vi "BAM Generation Create New TP Connection.vi"(5 "Data to Send":T1 {"Identifier" format="%08x"}, 11 "error in (no error)":errorcluster) -> (4 "Connection Cluster":T2 {"Packets"."Identifier" format="%08x"}, 6 "Connection Management Packet":T1 {"Identifier" format="%08x"}, 15 "error out":errorcluster)   [LabVIEW 2015, in "J1939 Addon Engine.lvlib"]
uses:
  J1939 Addon Engine.lvlib
  Types/BAM Generation Connection Cluster.ctl
  Shared/J1939 Utilities/Types/CAN Outgoing Message Cluster.ctl
  Shared/J1939 Utilities/SubVIs/TP.CM BAM.vi
  Shared/J1939 Utilities/SubVIs/TP.DT.vi
  Shared/J1939 Utilities/SubVIs/Convert CAN Arb ID to J1939 ID.vi
  Shared/J1939 Utilities/SubVIs/Convert J1939 ID to CAN Arb ID.vi
  Shared/J1939 Utilities/J1939 Utilities.lvlib
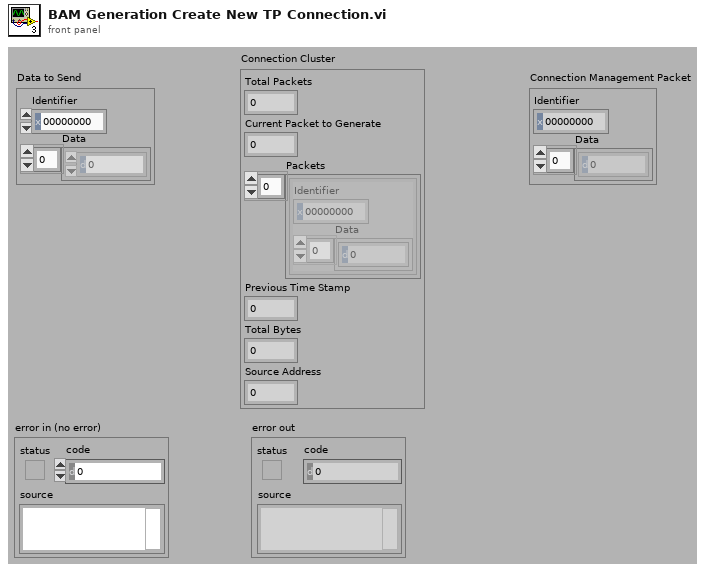
[diagram p1: front panel]
types:
  T1 = typedef "J1939 Addon Shared.lvlib/J1939 Utilities.lvlib/CAN Outgoing Message Cluster.ctl" = cluster{"Identifier":u32, "Data":u8[]}
  T2 = typedef "J1939 Addon Engine.lvlib/BAM Generation Connection Cluster.ctl" = cluster{"Total Packets":u8, "Current Packet to Generate":u8, "Packets":T1[], "Previous Time Stamp":u32, "Total Bytes":u16, "Source Address":u8}
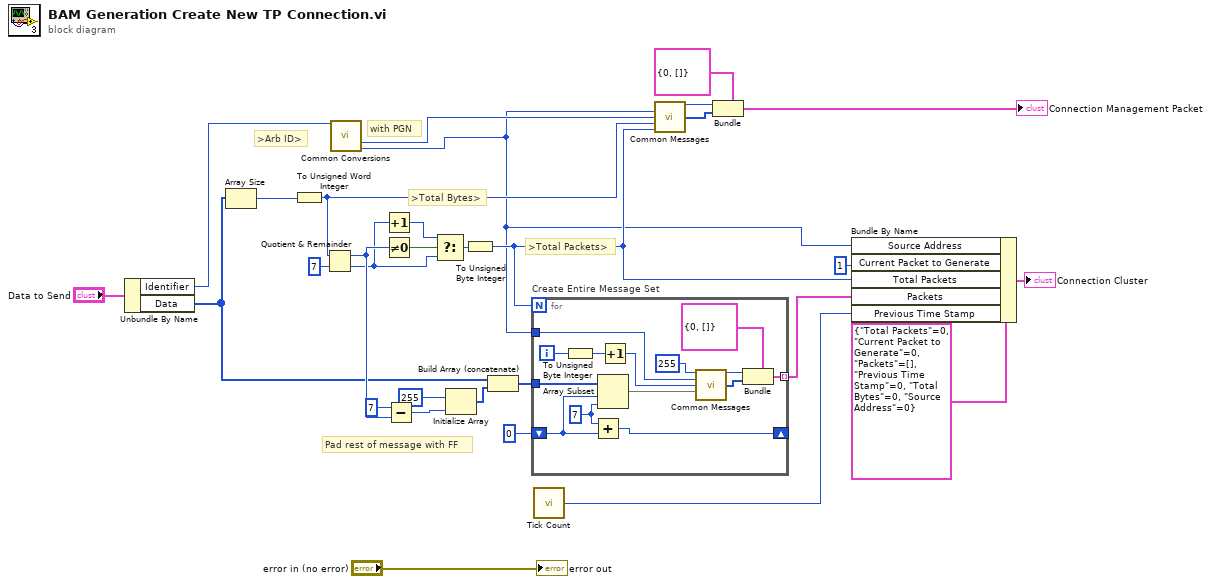
[diagram p0: block diagram]
diagram:
  # "Pad rest of message with FF"
  # ">Arb ID>"
  # "with PGN"
  # ">Total Packets>"
  # ">Total Bytes>"
  n1 = Unbundle By Name("Data to Send") -> ("Identifier"=w3:u32, "Data"=w5:u8[])
  n2 = Array Size(array=w5) -> (size(s)=w6:i32)
  n3 = To Unsigned Word Integer(number=w6) -> (unsigned 16bit integer=w12:u16)
  n4 = Quotient & Remainder(x=w12, y=u16 7) -> (x-y*floor(x/y)=w23:u16, floor(x/y)=w18:u16)
  n5 = call-poly "Common Conversions.vi"("Arb ID"=w3) -> ("PGN"=w2:u32, "Source Address"=w1:u8)  [unwired: 13 out]
  n6 = Increment(x=w18) -> (x+1=w17:u16)
  n7 = Not Equal To 0?(x=w23) -> (x != 0?=w16:bool)
  n8 = Subtract(x=u8 7, y=w23) -> (x-y=w25:u16)
  n9 = Select(t=w17, s=w16, f=w18) -> (s? t:f=w19:u16)
  n10 = Initialize Array(u8 255, w25) -> (w26:u8[])
  n11 = To Unsigned Byte Integer(number=w19) -> (unsigned 8bit integer=w28:u8)
  n12 = Build Array (concatenate)(w5, w26) -> (w27:u8[])
  n13 = for "Create Entire Message Set" {
    N: w28 -> [_]
    tunnel: w27 -> [w44]
    shift-right: [w41] -> _
    shift-left: 0 ("index") -> [w42]
    tunnel: [w33] -> w9 mode=indexing
    tunnel: w1 -> [w38]
    i -> [w40]
    w43 = 7 ("length")
    n14 = To Unsigned Byte Integer(number=w40) -> (unsigned 8bit integer=w39:u8)
    n15 = Add(x=w43, y=w42) -> (x+y=w41:i32)
    n16 = Array Subset(array=w44, index=w42, length=w43) -> (w32:u8[])
    n17 = Increment(x=w39) -> (x+1=w37:u8)
    n18 = call-poly "Common Messages.vi"("Destination Address"=u8 255, "Source Address"=w38, "Sequence Number"=w37, "Data"=w32) -> ("Arb ID"=w35:u32, "Data"=w34:u8[])  [unwired: 10 out]
    n19 = Bundle(cluster=T1 {"Identifier"=0, "Data"=[]}, "Identifier"=w35, "Data"=w34) -> (w33:T1)
  }
  n20 = call "Tick Count"() -> ("Tick Count(mSec)"=w10:u32)
  n21 = call-poly "Common Messages.vi"("Source Address"=w1, "PGN"=w2, "Total Message Size(bytes)"=w12, "Total Number of Packets"=w28) -> ("Arb ID"=w29:u32, "Data"=w30:u8[])  [unwired: 10 out]
  n22 = Bundle(cluster=T1 {"Identifier"=0, "Data"=[]}, "Identifier"=w29, "Data"=w30) -> (→"Connection Management Packet":T1)
  n23 = Bundle By Name(cluster=T2 {"Total Packets"=0, "Current Packet to Generate"=0, "Packets"=[], "Previous Time Stamp"=0, "Total Bytes"=0, "Source Address"=0} ("Cluster"), "Source Address"=w1, "Current Packet to Generate"=u8 1, "Total Packets"=w28, "Packets"=w9, "Previous Time Stamp"=w10) -> (→"Connection Cluster":T2)
  "error out" <- "error in (no error)"
